vi "Set Front Panel Object Control Value.vi"(8 "error in":errorcluster, 10 "Control (F: Indicator)":bool=TRUE, 11 "vi reference":refnum<vi>) -> (0 "error out":errorcluster, 1 "Found?":bool, 2 "Control Value":cluster{"name":string, "value":variant}, 3 "dup vi reference":refnum<vi>)   [LabVIEW 2013, in "VITesterUtilities.lvlib"]
doc: "Sets the FP control value of an LVClass control, whose type matches the specific type of object in <B>Object in</B> to the value of <B>Object in</B>."
uses:
  Libraries/VITesterUtilities.lvlib
  Classes/TestCase/TestCase.lvclass
  JKI Reuse/Is an Error (error cluster)__jki_lib_error_handling -- VI Tester.vi
panel:
  # "Copyright © 2007 James Kring, Inc. All rights reserved.\n\nAuthor: Jim Kring <jim.kring@jameskring.com>\n\nThis library is provided \"AS IS\" , WITHOUT WARRANTIES OR \nCONDITIONS OF ANY KIND, either express or implied.\n\nJames Kring, Inc. -- http://www.jameskring.com"
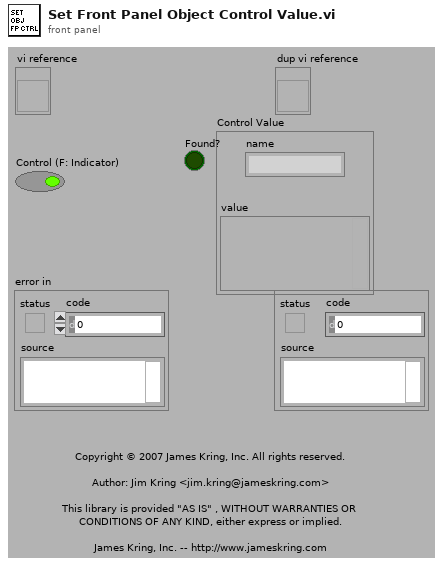
[diagram p1: front panel]
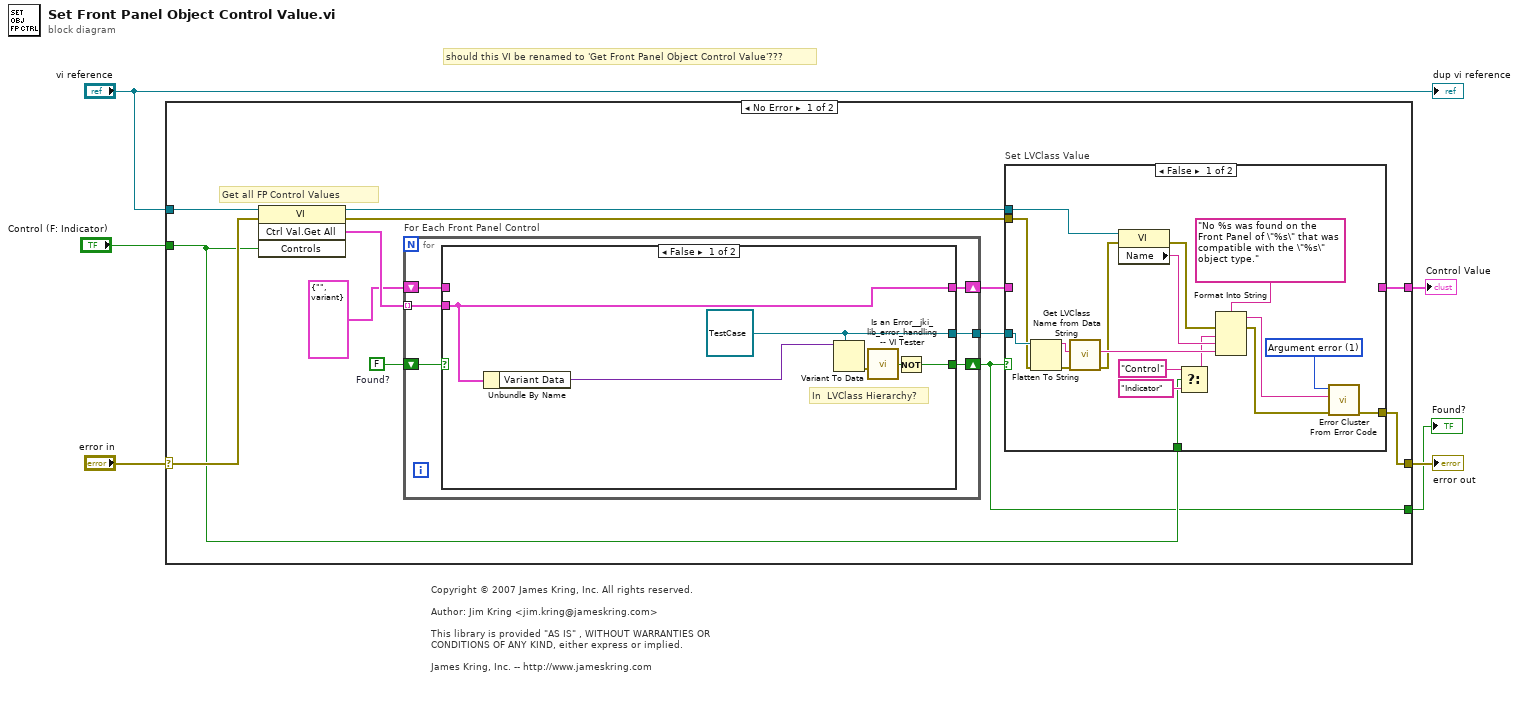
[diagram p0: block diagram]
diagram:
  # "should this VI be renamed to 'Get Front Panel Object Control Value'???"
  # "Copyright © 2007 James Kring, Inc. All rights reserved.\n\nAuthor: Jim Kring <jim.kring@jameskring.com>\n\nThis library is provided \"AS IS\" , WITHOUT WARRANTIES OR \nCONDITIONS OF ANY KIND, either express or implied.\n\nJames Kring, Inc. -- http://www.jameskring.com"
  n1 = case shown="No Error" "error in" {
    selector: "error in" -> [w13 w54]
    tunnel: [w19 w54] -> w5
    tunnel: "vi reference" -> [w17 _]
    tunnel: "Control (F: Indicator)" -> [w10 _]
    tunnel: [w9 _] -> w2
    tunnel: [w8 _] -> w1
    frame No Error {
      w14 = FALSE  # Found?
      # "Get all FP Control Values"
      n2 = invoke class="VI" method="Ctrl Val.Get All"(reference=w17, error in=w13, "Controls"=w10) -> (reference out=w18:refnum<vi>, error out=w16:errorcluster, "Get All Control Values Variant"=w15:cluster{"Name":string, "Variant Data":variant}[])  [unwired: 1 in, 1 out]
      n3 = for "For Each Front Panel Control" {
        tunnel: w15 -> [w24] mode=indexing
        shift-right: [w25] -> w8
        shift-left: w14 -> [w23]
        shift-right: [w22] -> w12
        shift-left: cluster{"name":string, "Value":variant} {"name"="", "Value"=variant} -> [w21]
        tunnel: [w20] -> w7
        n4 = case shown="False" w23 {
          selector: w23 -> [_ w33]
          tunnel: [w31 w33] -> w25
          tunnel: w24 -> [w30 _]
          tunnel: [w30 w32] -> w22
          tunnel: w21 -> [_ w32]
          tunnel: [w26 _] -> w20
          frame False {
            w26 = refnum<class "TestCase.lvclass"> refnum ("TestCase.lvclass")
            # "In  LVClass Hierarchy?"
            n5 = Unbundle By Name(w30) -> ("Variant Data"=w27:variant)
            n6 = Variant To Data(type=w26, Variant=w27) -> (error out=w28:errorcluster)  [unwired: 1 in, 1 out]
            n7 = call-poly "Is an Error__jki_lib_error_handling -- VI Tester.vi"("error in"=w28) -> ("error?"=w29:bool)  [unwired: 8 in]
            n8 = Not(x=w29) -> (.not. x?=w31:bool)
          }
          frame True {
          }
        }
      }
      n9 = case "Set LVClass Value" shown="False" w8 {
        tunnel: w12 -> [_ w53]
        tunnel: [w51 w52] -> w19
        tunnel: w18 -> [w49 _]
        tunnel: w16 -> [w34 w52]
        tunnel: w10 -> [w39 _]
        tunnel: [_ w53] -> w9
        tunnel: w7 -> [w37 _]
        frame False {
          w50 = 1 items=["No error", "Argument error", "Memory is full", "Out of zone", "End of file", "File already open", "Generic file I/O error", "File not found", "File permission error", "Disk is full", "Duplicate path", "Too many files open", "System feature not enabled", "Resource file not found", "Cannot add resource", "Resource not found", "Image not found", "Image memory error", "Pen does not exist", "Config type invalid", "Config token not found", "Config parse error", "Config memory error", "Bad external code format", "Bad external code offset", "External code not present", "Null window", "Destroy window error", "Null menu", "Print aborted", "Bad print record", "Print driver error", "Windows error during printing", "Memory error during printing", "Print dialog error", "Generic print error", "Invalid device refnum", "Device not found", "Device parameter error", "Device unit error", "Cannot open device", "Device call aborted", "Generic error", "Cancelled by user", "Object ID too low", "Object ID too high", "Object not in heap", "Unknown heap", "Unknown object (invalid DefProc)", "Unknown object (DefProc not in table)", "Message out of range", "Invalid (null) method", "Unknown message", "Manager call not supported", "Bad address", "Network operation in progress", "Network operation timed out", "Connection is busy", "Network attribute not supported", "Network error", "Address in use", "System out of memory", "Connection aborted", "Connection refused", "Not connected", "Already connected", "Connection closed", "Initialization error (interapplication manager)", "Bad occurrence", "Wait on unbound occurrence handler", "Occurrence queue overflow", "Datalog type conflict", "Unused", "Unrecognized type (interapplication manager)", "Memory corrupt", "Failed to make temporary DLL", "Old CIN version", "Drag socket not found", "Failed to load drop-object", "Failed to register OLE object", "Failed to release OLE object", "Format specifier type mismatch", "Unknown format specifier", "Too few format specifiers", "Too many format specifiers", "Scan failed", "Newer CIN version", "Error converting to variant", "Runtime menu error", "Password tampered", "Variant attribute not found", "Incompatible variant data type", "Event data is not available", "Event Store is not present", "Occurrence is not found", "Event Queue is not created", "Event info is not available", "Refnum passed is NULL", "Error retrieving Class GUID", "Error retrieving CoClass GUID", "Error retrieving TypeLib GUID.", "Bad built application magic bytes.", "Specific driver is different from the specific driver associated with the Logical Name.", "There is no session opened to the class driver.", "Max Error", "MAX - Error with config objects", "MAX - Error loading configuration", "MAX - Group not supported"]
          n10 = Flatten To String(anything=w37, error in (no error)=w34) -> (data string=w36:string, error out=w35:errorcluster)  [unwired: 2 in, 1 out]
          n11 = call "Get LVClass Name from Data String.vi"("error in"=w35, "LVClass Data String"=w36) -> ("error out"=w43:errorcluster, "LVClass Name"=w44:string)  [unwired: 8 in]
          n12 = property class="VI"(reference=w49, error in=w43) -> (error out=w46:errorcluster, "Name"=w48:string)  [unwired: 1 out]
          n13 = Select(t="Control", s=w39, f="Indicator") -> (s? t:f=w42:string)
          n14 = Format Into String(format string="No %s was found on the Front Panel of \"%s\" that was compatible with the \"%s\" object type.", error in=w46, w42, w48, w44) -> (resulting string=w38:string, error out=w45:errorcluster)  [unwired: 1 in]
          n15 = call <vilib>:"Error Cluster From Error Code.vi"("error in (no error)"=w45, "error message (\"\")"=w38, "error code (0)"=w50) -> ("error out"=w51:errorcluster)  [unwired: 6 in]
        }
        frame True {
        }
      }
    }
    frame Error {
    }
  }
  "error out" <- w5
  "Control Value" <- w2
  "Found?" <- w1
  "dup vi reference" <- "vi reference"
